vi "GDSProject_RemoveFullyQualifiedNamesIfPossible.vi"(11 "ItemnamesIn":string[](array[string])) -> (3 "ItemnamesOut":string[](array[string]))   [LabVIEW 2020]
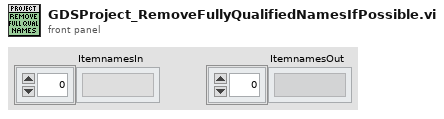
[diagram p1: front panel]
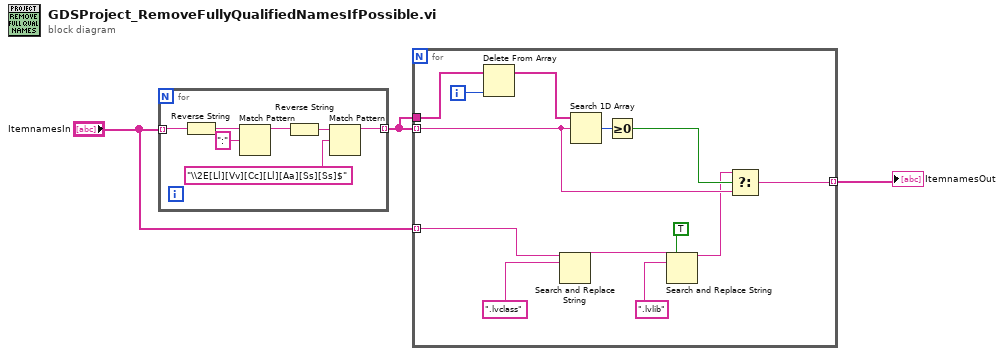
[diagram p0: block diagram]
diagram:
  n1 = for {
    tunnel: "ItemnamesIn" -> [w10] mode=indexing
    tunnel: [w4] -> w1 mode=indexing
    n2 = Reverse String(1:w10) -> (0:w9:string)
    n3 = Match Pattern(string=w9, regular expression=":") -> (before substring=w7:string)  [unwired: 1 in, 3 out]
    n4 = Reverse String(1:w7) -> (0:w5:string)
    n5 = Match Pattern(string=w5, regular expression="\\2E[Ll][Vv][Cc][Ll][Aa][Ss][Ss]$") -> (before substring=w4:string)  [unwired: 1 in, 3 out]
  }
  n6 = for {
    tunnel: w1 -> [w21] mode=indexing
    tunnel: w1 -> [w19]
    tunnel: "ItemnamesIn" -> [w12] mode=indexing
    tunnel: [w20] -> w3 mode=indexing
    i -> [w17]
    n7 = Delete From Array(array=w19, index=w17) -> (array with subset deleted=w18:string[])  [unwired: 1 in, 1 out]
    n8 = Search and Replace String(input string=w12, search string=".lvclass" ("regular expression")) -> (result string=w13:string)  [unwired: 6 in, 3 out]
    n9 = Search 1D Array(1D array=w18, element=w21) -> (index of element=w23:i32)  [unwired: 1 in]
    n10 = Greater Or Equal To 0?(x=w23) -> (x >= 0?=w22:bool)
    n11 = Search and Replace String(replace all?=TRUE ("replace all? (F)"), input string=w13, search string=".lvlib" ("regular expression")) -> (result string=w14:string)  [unwired: 5 in, 3 out]
    n12 = Select(t=w14, s=w22, f=w21) -> (s? t:f=w20:string)
  }
  "ItemnamesOut" <- w3
